vi "dist_2_points.vi"(10 "point in 2":cluster{"x":dbl, "y":dbl}, 11 "point in 1":cluster{"x":dbl, "y":dbl}) -> (3 "distance":dbl)   [LabVIEW 2016]
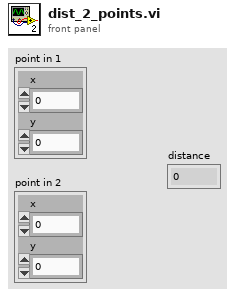
[diagram p1: front panel]
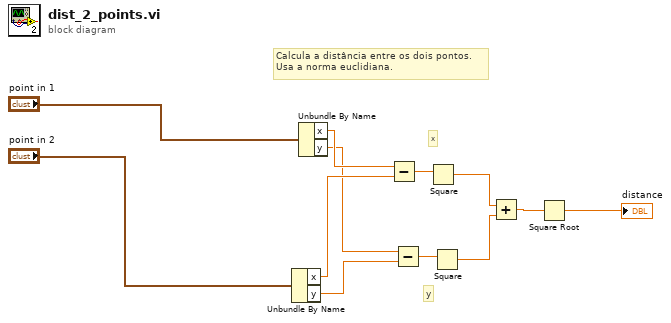
[diagram p0: block diagram]
diagram:
  # "y"
  # "x"
  # "Calcula a distância entre os dois pontos.\nUsa a norma euclidiana."
  n1 = Unbundle By Name("point in 2") -> ("x"=w9:dbl, "y"=w2:dbl)
  n2 = Unbundle By Name("point in 1") -> ("x"=w10:dbl, "y"=w3:dbl)
  n3 = Subtract(x=w10, y=w9) -> (x-y=w8:dbl)
  n4 = Subtract(x=w3, y=w2) -> (x-y=w4:dbl)
  n5 = Square(x=w8) -> (x^2=w7:dbl)
  n6 = Square(x=w4) -> (x^2=w1:dbl)
  n7 = Add(x=w7, y=w1) -> (x+y=w6:dbl)
  n8 = Square Root(x=w6) -> (sqrt(x)=→"distance":dbl)
